vi "Read Results from processing.vi"(8 "error in":errorcluster, 11 "Tank Controller Logic runtime in":refnum<class "Tank Controller Logic runtime.lvclass">) -> (0 "error out":errorcluster, 2 "Results from processing":T1, 3 "Tank Controller Logic runtime out":refnum<class "Tank Controller Logic runtime.lvclass">)   [LabVIEW 2017, in "Tank Controller Logic runtime.lvclass"]
uses:
  Tank Controller Logic runtime.lvclass
  configuration/result data indices.ctl
  Tank Controller Logic runtime.lvclass/Tank Controller Logic runtime.ctl
  configuration/Tank Controller Logic configuration.lvclass
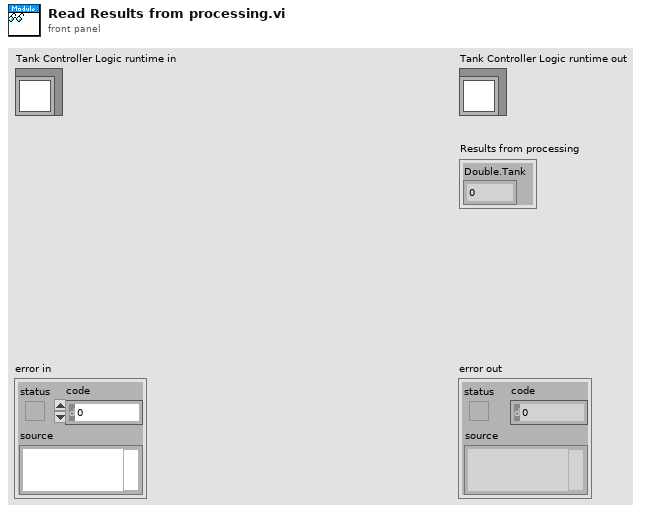
[diagram p1: front panel]
types:
  T1 = typedef "Tank Controller Logic configuration.lvclass/result data indices.ctl" = cluster{"Double.Tank":i32}
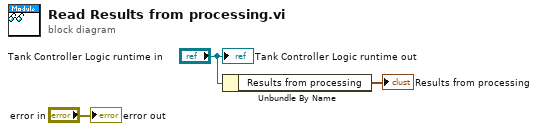
[diagram p0: block diagram]
diagram:
  n1 = Unbundle By Name("Tank Controller Logic runtime in") -> ("Results from processing"=→"Results from processing":T1)
  "error out" <- "error in"
  "Tank Controller Logic runtime out" <- "Tank Controller Logic runtime in"
